vi "UTILITY Create Plot Array.vi"(8 "Error In":errorcluster, 10 "Save Data":string[][](array[string]), 11 "Plot Array in":dbl[][](array[numeric])) -> (0 "Error Out":errorcluster, 3 "Plot Array out":dbl[][](array[numeric]))   [LabVIEW 2018]
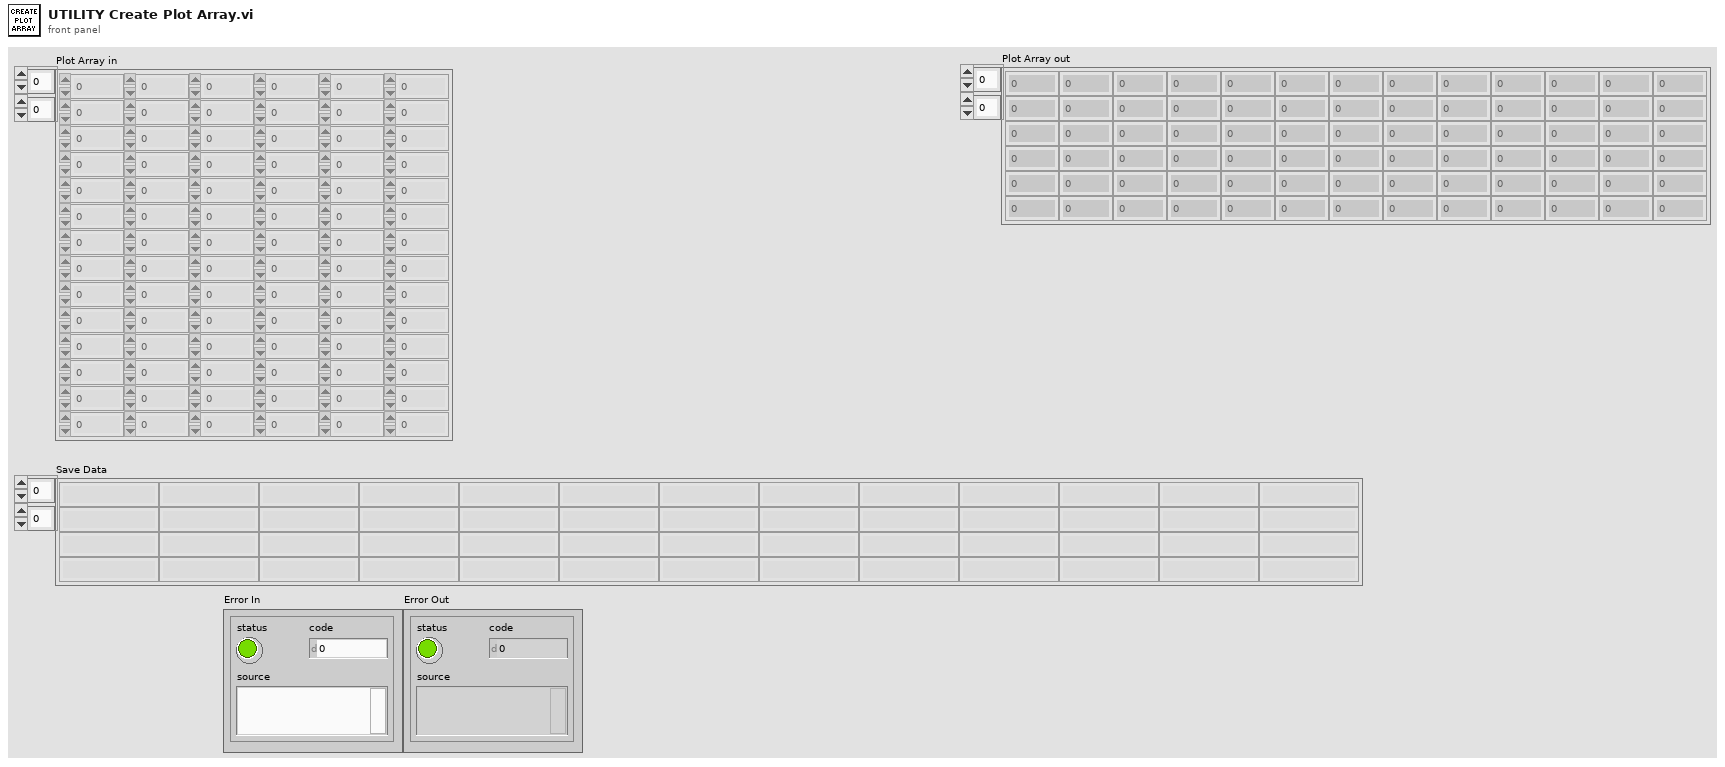
[diagram p1: front panel]
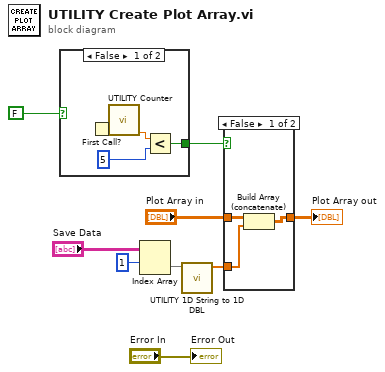
[diagram p0: block diagram]
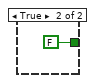
[diagram p2: hidden frame]
diagram:
  n1 = case shown="False" FALSE {
    tunnel: [w11 FALSE] -> w8
    frame False {
      n2 = First Call?() -> (First Call?: T/F=w13:bool)
      n3 = call "UTILITY Counter.vi"("Reset"=w13) -> ("Count"=w12:dbl)  [unwired: 10 in]
      n4 = Less?(x=w12, y=5) -> (x < y?=w11:bool)
    }
    frame True {
    }
  }
  n5 = Index Array(array="Save Data", index (row)=1 ("disabled index (col)")) -> (element=w5:string[])  [unwired: 1 in]
  n6 = call "UTILITY 1D String to 1D DBL.vi"("Save Data"=w5) -> ("DBL"=w6:dbl[])  [unwired: 10 in]
  n7 = case shown="False" w8 {
    tunnel: w6 -> [w15 _]
    tunnel: [w17 w18] -> w9
    tunnel: "Plot Array in" -> [w16 w18]
    frame False {
      n8 = Build Array (concatenate)(w16, w15) -> (w17:dbl[][])
    }
    frame True {
    }
  }
  "Plot Array out" <- w9
  "Error Out" <- "Error In"
